vi "Multiple Transducers_XiaoyeV4.vi"() -> ()   [LabVIEW 2022 SP3]
doc: "Reads force and torque values from multiple ATI transducers."
uses:
  <vilib>/DAQmx/read.llb/DAQmx Read (Analog 2D DBL NChan NSamp).vi
  <vilib>/Analysis/baseanly.llb/A x Vector.vi
  <vilib>/DAQmx/create/channels.llb/DAQmx Create Channel (AI-Voltage-Basic).vi
  <vilib>/DAQmx/configure/timing.llb/DAQmx Timing (Sample Clock).vi
  <vilib>/DAQmx/configure/trigger.llb/DAQmx Start Trigger (Digital Edge).vi
  <vilib>/DAQmx/miscellaneous.llb/DAQmx Fill In Error Info.vi
  <vilib>/Analysis/NI_AALBase.lvlib
panel:
  in  "User Torque Units":string
  in  "User Force Units":string
  in  "Calibration Units":T1(array[cluster])
  in  "Tool Transforms":T2(array[cluster])
  in  "Scan Lists":string[](array[string])=["dev1/ai0:5,dev1/ai6:11"]
  in  "Enable Transducer":bool[](array[boolean])
  in  "Filename":path=path "C:/Users/admin/Desktop/迎辉软件/2021Multiple Transducers 文件夹(1)/保存文件/231423143.csv"
  in  "Connection Mode":i32(ring)=-1 items=["default"=-1, "RSE"=10083, "NRSE"=10078, "Differential"=10106, "Pseudodifferential"=12529]
  in  "Bias All":bool
  in  "Start Saving Data":bool
  in  "Bias Transducer":bool[](array[boolean])
  in  "Append Data?":bool
  in  "Samples to Read at a time":i32=50
  out "Voltages":dbl[][](array[numeric])
  in  "Buffer Size":i32=1000
  in  "Sample Rate":dbl=1000.0
  out "F/T Values":dbl[][][](array[numeric])
  in  "Calibration Files":path[](array[path])=[path "C:/Program Files/ATI DAQ FT/FT5816.cal", path "C:/Program Files/ATI DAQ FT/FT5395.cal"]
  # "dev2/ai0:5,dev2/ai16:21"
  # "For assistance, turn on context help and examine\nthe help text for each control."
  # "Fx"
  # "Fy"
  # "Fz"
  # "Tx"
  # "Ty"
  # "Tz"
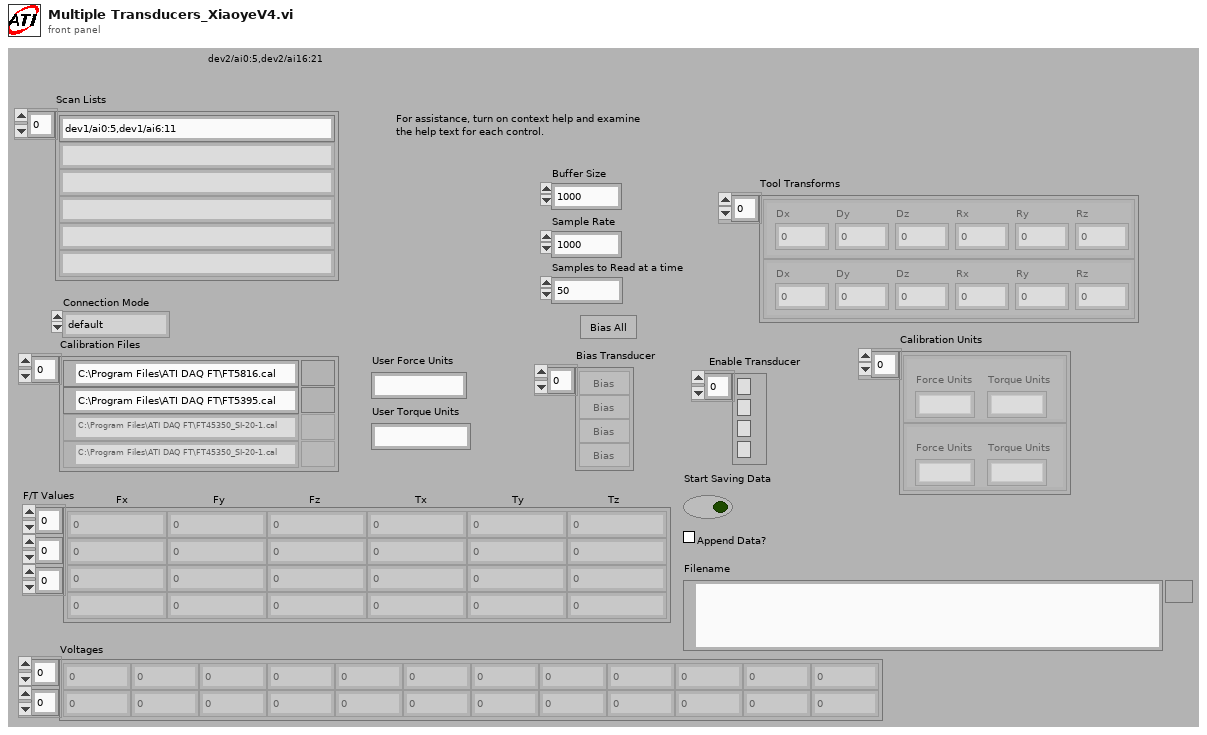
[diagram p1: front panel]
types:
  T1 = cluster{"Force Units":string, "Torque Units":string}[]
  T2 = cluster{"Dx":dbl, "Dy":dbl, "Dz":dbl, "Rx":dbl, "Ry":dbl, "Rz":dbl}[]
  T3 = cluster{"Calibration Force Units":string, "Calibration Torque Units":string}
  T4 = enum16{"open", "open or create", "create or replace", "create", "open (read only)"}
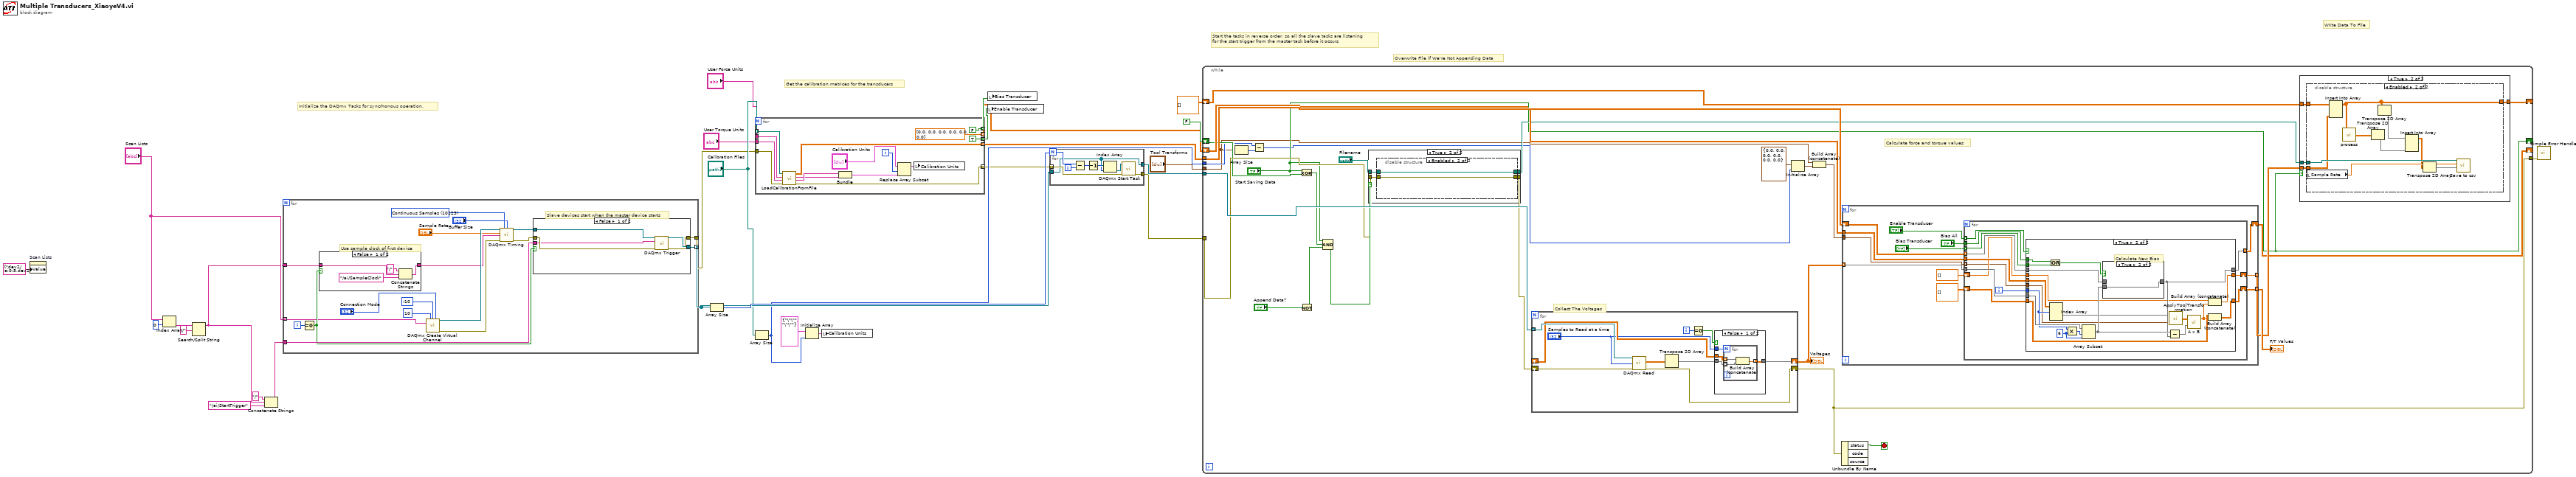
[diagram p0: block diagram]
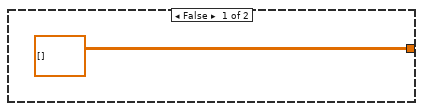
[diagram p2: hidden frame]
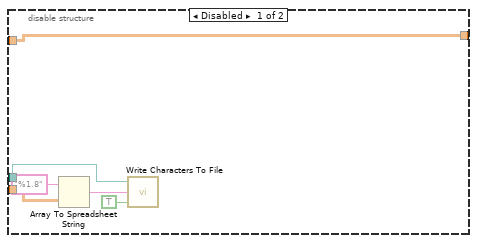
[diagram p3: hidden frame]
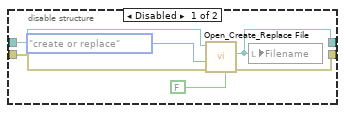
[diagram p5: hidden frame]
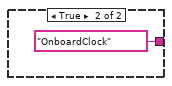
[diagram p9: hidden frame]
diagram:
  # "Overwrite File if We're Not Appending Data"
  # "Write Data To File"
  # "Initialize the DAQmx Tasks for syncrhonous operation."
  # "Get the calibration matrices for the transducers"
  # "Start the tasks in reverse order, so all the slave tasks are listening \nfor the start trigger from the master task before it occurs"
  n1 = property on="Scan Lists" class="Arr (strict)"("Value"=string[] ["dev2/ai0:5,dev2/ai16:21"] ("Scan Lists")) -> ()  [unwired: 2 in, 2 out]
  n2 = Index Array(array="Scan Lists", index=0) -> (element=w16:string)
  n3 = Search/Split String(string=w16, search string/char (-)="/") -> (substring before match=w14:string)  [unwired: 1 in, 2 out]
  n4 = Concatenate Strings("/", w14, "/ai/StartTrigger") -> (w28:string)
  n5 = for {
    tunnel: w28 -> [w41]
    tunnel: [w38] -> w4
    tunnel: [w32] -> w19 mode=indexing
    tunnel: "Scan Lists" -> [w31] mode=indexing
    tunnel: w14 -> [w30]
    i -> [w43]
    w45 = 10123 items=["Finite Samples"=10178, "Continuous Samples"=10123, "Hardware Timed Single Point"=12522] ("sample mode")
    # "Slave devices start when the master device starts"
    # "Use sample clock of first device"
    n6 = Equal To 0?(x=w43) -> (x = 0?=w37:bool)
    n7 = case shown="False" w37 {
      tunnel: [w49 tag "OnboardClock"] -> w36
      tunnel: w30 -> [w48 _]
      frame False {
        n8 = Concatenate Strings("/", w48, "/ai/SampleClock") -> (w49:string)
      }
      frame True {
      }
    }
    n9 = call-poly <vilib>:"DAQmx Create Virtual Channel.vi"("maximum value"=10, "minimum value"=-10, "input terminal configuration"="Connection Mode", "physical channels"=w31) -> ("task out"=w47:refnum<k21>, "error out"=w40:errorcluster)  [unwired: 10 in]
    n10 = call-poly <vilib>:"DAQmx Timing.vi"("task/channels in"=w47, "sample mode"=w45, "samples per channel"="Buffer Size", "rate"="Sample Rate", "source"=w36, "error in"=w40) -> ("task out"=w42:refnum<k21>, "error out"=w39:errorcluster)  [unwired: 8 in]
    n11 = case shown="False" w37 {
      tunnel: w42 -> [w57 w59]
      tunnel: [w56 w59] -> w32
      tunnel: w41 -> [w53 _]
      tunnel: w39 -> [w55 w58]
      tunnel: [w54 w58] -> w38
      frame False {
        n12 = call-poly <vilib>:"DAQmx Trigger.vi"("task/channels in"=w57, "source"=w53, "error in"=w55) -> ("task out"=w56:refnum<k21>, "error out"=w54:errorcluster)  [unwired: 11 in]
      }
      frame True {
      }
    }
  }
  n13 = Array Size(array=w19) -> (size(s)=w21:i32)
  n14 = for {
    tunnel: "Calibration Files" -> [w72] mode=indexing
    tunnel: [FALSE] -> w25 mode=indexing
    tunnel: [TRUE] -> w23 mode=indexing
    tunnel: [w70] -> w22 mode=indexing
    tunnel: [dbl[] [0.0, 0.0, 0.0, 0.0, 0.0, 0.0]] -> w12 mode=indexing
    tunnel: "User Force Units" -> [w63]
    tunnel: "User Torque Units" -> [w62]
    tunnel: w4 -> [w61]
    tunnel: [w60] -> w3 mode=indexing
    i -> [w69]
    n15 = call "LoadCalibrationFromFile.vi"("Error In"=w61, "User Torque Units"=w62, "User Force Units"=w63, "Cal File Path"=w72) -> ("Error Out"=w60:errorcluster, "Calibration Force Units"=w66:string, "Calibration Torque Units"=w65:string, "Calibration Matrix"=w70:dbl[][])
    n16 = Bundle("Calibration Force Units"=w66, "Calibration Torque Units"=w65) -> (w67:T3)  [unwired: 1 in]
    n17 = Replace Array Subset(array="Calibration Units", new element=w67, index=w69) -> (w64:T1)
    n18 = local write "Calibration Units"(w64) -> ()
  }
  n19 = Array Size(array="Calibration Files") -> (size(s)=w8:i32)
  n20 = Initialize Array(cluster{string, string} {"\"\"", "\"\""}, w8) -> (w7:cluster{string, string}[])
  n21 = local write "Calibration Units"(w7) -> ()
  n22 = local write "Enable Transducer"(w23) -> ()
  n23 = local write "Bias Transducer"(w25) -> ()
  n24 = for {
    N: w21 -> [w82]
    tunnel: w19 -> [w77]
    tunnel: w3 -> [w78] mode=indexing
    tunnel: [w77] -> w27
    tunnel: [w75] -> w13
    i -> [w81]
    n25 = Subtract(x=w82, y=w81) -> (x-y=w80:i32)
    n26 = Decrement(x=w80) -> (x-1=w76:i32)
    n27 = Index Array(array=w77, index=w76) -> (element=w79:refnum<k21>)
    n28 = call <vilib>:"DAQmx Start Task.vi"("task/channels in"=w79, "error in"=w78) -> ("error out"=w75:errorcluster)  [unwired: 12 in, 1 out]
  }
  n29 = while {
    tunnel: w27 -> [w110]
    tunnel: w22 -> [w108]
    shift-right: [w97] -> _
    shift-left: w12 -> [w106]
    shift-right: ["Start Saving Data"] -> _
    shift-left: FALSE -> [w96]
    tunnel: w13 -> [w100]
    tunnel: [w92] -> w20
    tunnel: "Tool Transforms" -> [w87]
    tunnel: w8 -> [w90]
    shift-right: [w84] -> _
    shift-left: dbl[][] [] -> [w83]
    stop <- w93 stop-if-true
    # "Calculate force and torque values"
    # "Collect The Voltages"
    n30 = Array Size(array=w87) -> (size(s)=w89:i32)
    n31 = Subtract(x=w90, y=w89) -> (x-y=w88:i32)
    n32 = Exclusive Or(1:w96, 2:"Start Saving Data") -> (0:w95:bool)
    n33 = Not(x="Append Data?") -> (.not. x?=w102:bool)
    n34 = Compound Arithmetic op=AND("Start Saving Data", w95, w102) -> (w105:bool)
    n35 = case shown="True" w105 {
      tunnel: "Filename" -> [w133 w137]
      tunnel: [w133 w134] -> w101
      tunnel: w100 -> [w132 w136]
      tunnel: [w132 w135] -> w99
      frame False {
      }
      frame True {
        n36 = disable-structure shown="Enabled" {
          disable-tunnel: w137 -> [w143 w145]
          disable-tunnel: w136 -> [w142 w144]
          disable-tunnel: [w141 w144] -> w135
          disable-tunnel: [w138 w145] -> w134
          frame Disabled {
            n37 = call <vilib>:"Open_Create_Replace File.vi"("advisory dialog? (display:T)"=FALSE, "error in (no error)"=w142, "function (open:0)"=T4."create or replace", "file path"=w143) -> ("error out"=w141:errorcluster, "new file path"=w138:path)  [unwired: 4 in, 2 out]
            n38 = local write "Filename"(w138) -> ()
          }
          frame Enabled {
          }
        }
      }
    }
    n39 = for {
      tunnel: w110 -> [w205] mode=indexing
      shift-right: [w202] -> w92
      shift-left: w99 -> [w204]
      shift-right: [w199] -> w109
      shift-left: _ -> [w197]
      i -> [w201]
      n40 = call-poly <vilib>:"DAQmx Read.vi"("task/channels in"=w205, "number of samples per channel"="Samples to Read at a time", "error in"=w204) -> ("data"=w203:dbl[][], "error out"=w202:errorcluster)  [unwired: 10 in, 1 out]
      n41 = Transpose 2D Array(2D array=w203) -> (transposed array=w198:dbl[][])
      n42 = Equal To 0?(x=w201) -> (x = 0?=w200:bool)
      n43 = case shown="False" w200 {
        tunnel: [w207 w213] -> w199
        tunnel: w198 -> [w208 w213]
        tunnel: w197 -> [w209 _]
        tunnel: "Samples to Read at a time" -> [w206 _]
        frame False {
          n44 = for {
            N: w206 -> [_]
            tunnel: w209 -> [w212] mode=indexing
            tunnel: w208 -> [w211] mode=indexing
            tunnel: [w210] -> w207 mode=indexing
            n45 = Build Array (concatenate)(w212, w211) -> (w210:dbl[])
          }
        }
        frame True {
        }
      }
    }
    "Voltages" <- w109
    n46 = Initialize Array(cluster{dbl, dbl, dbl, dbl, dbl, dbl} {0.0, 0.0, 0.0, 0.0, 0.0, 0.0}, w88) -> (w86:cluster{dbl, dbl, dbl, dbl, dbl, dbl}[])
    n47 = Build Array (concatenate)(w87, w86) -> (w85:T2)
    n48 = Unbundle By Name(w92) -> ("status"=w93:bool)  [unwired: 2 out]
    n49 = for {
      tunnel: w109 -> [w156] mode=indexing
      tunnel: w108 -> [w157]
      tunnel: [w147] -> w107 mode=indexing
      tunnel: [w152] -> w98 mode=indexing
      shift-right: [w150] -> w97
      shift-left: w106 -> [w155]
      tunnel: w85 -> [w146]
      n50 = for {
        tunnel: w157 -> [w165]
        tunnel: w156 -> [w170]
        tunnel: w155 -> [w168] mode=indexing
        tunnel: "Bias Transducer" -> [w169] mode=indexing
        tunnel: [w167] -> w150 mode=indexing
        shift-right: [w162] -> w152
        shift-left: dbl[] [] -> [w163]
        tunnel: "Bias All" -> [w166]
        tunnel: "Enable Transducer" -> [w161] mode=indexing
        shift-right: [w159] -> w147
        shift-left: sgl[][] [] -> [w160]
        tunnel: w146 -> [w158] mode=indexing
        i -> [w164]
        n51 = case shown="True" w161 {
          tunnel: w170 -> [_ w191]
          tunnel: w169 -> [_ w190]
          tunnel: w168 -> [w173 w188]
          tunnel: [w173 w186] -> w167
          tunnel: w166 -> [_ w184]
          tunnel: w165 -> [_ w183]
          tunnel: w164 -> [_ w182]
          tunnel: w163 -> [w172 w181]
          tunnel: [w172 w180] -> w162
          tunnel: w160 -> [w171 w179]
          tunnel: [w171 w177] -> w159
          tunnel: w158 -> [_ w175]
          frame False {
          }
          frame True {
            w192 = 6
            # "Calculate New Bias"
            n52 = Or(x=w184, y=w190) -> (x .or. y?=w189:bool)
            n53 = Index Array(array=w183, index (dim 0)=w182) -> (element=w176:dbl[][])  [unwired: 2 in]
            n54 = Multiply(x=w182, y=w192) -> (x*y=w193:i32)
            n55 = Array Subset(array=w191, index=w193, length=w192) -> (w187:dbl[])
            n56 = case shown="True" w189 {
              tunnel: w187 -> [_ w195]
              tunnel: [w194 w195] -> w186
              tunnel: w188 -> [w194 _]
              frame False {
              }
              frame True {
              }
            }
            n57 = Subtract(x=w187, y=w186) -> (x-y=w185:dbl[])
            n58 = call "ApplyToolTransformation.vi"("Transform"=w175, "Calibration Matrix"=w176) -> ("Transformed Calibration Matrix"=w174:dbl[][])
            n59 = call-poly <vilib>:"A x B.vi"("Vector"=w185, "A"=w174) -> ("A x Vector"=w178:dbl[])  [unwired: 1 out]
            n60 = Build Array (concatenate)(w181, w178) -> (w180:dbl[])
            n61 = Build Array (concatenate)(w179, w178) -> (w177:dbl[][])
          }
        }
      }
    }
    "F/T Values" <- w107
    n62 = case shown="True" "Start Saving Data" {
      tunnel: w101 -> [_ w115]
      tunnel: w98 -> [_ w114]
      tunnel: [dbl[][] [] w113] -> w84
      tunnel: w83 -> [_ w112]
      frame False {
      }
      frame True {
        n63 = disable-structure shown="Enabled" {
          disable-tunnel: w115 -> [w121 w131]
          disable-tunnel: w114 -> [w118 w129]
          disable-tunnel: [w116 w127] -> w113
          disable-tunnel: w112 -> [w116 w128]
          frame Disabled {
            n64 = Array To Spreadsheet String(array=w118, 3:"%1.8" ("format string")) -> (spreadsheet string=w117:string)  [unwired: 1 in]
            n65 = call <vilib>:"Write Characters To File.vi"("append to file? (new file:F)"=TRUE, "character string"=w117, "file path (dialog if empty)"=w121) -> ()  [unwired: 2 in, 1 out]
          }
          frame Enabled {
            n66 = local read "Sample Rate"() -> (w130:dbl)
            n67 = Insert Into Array(array=w128, new element=w129) -> (w127:dbl[][])  [unwired: 2 in]
            n68 = call "process.vi"("input"=w127) -> ("xxxx"=w126:dbl[][])
            n69 = Transpose 2D Array(2D array=w126) -> (transposed array=w124:dbl[][])
            n70 = Transpose 2D Array(2D array=w127) -> (transposed array=w123:dbl[][])
            n71 = Insert Into Array(array=w123, new element=w124) -> (w125:dbl[][])  [unwired: 2 in]
            n72 = Transpose 2D Array(2D array=w125) -> (transposed array=w122:dbl[][])
            n73 = call "Save to csv.vi"("Array"=w122, "Rate"=w130, "file path (dialog if empty)"=w131) -> ()  [unwired: 8 in, 1 out]
          }
        }
      }
    }
  }
  n74 = call <vilib>:"Simple Error Handler.vi"("error in (no error)"=w20) -> ()  [unwired: 4 in, 5 out]
